vi "校准信息解析.vi"(11 "校准信息":u16[](array[numeric]) caption="关键参数") -> ()   [LabVIEW 2016, in "数据传输系统-02.lvlib"]
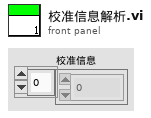
[diagram p1: front panel]
types:
  T1 = cluster{"低标液1浓度":dbl, "低标液1信号值":dbl, "低标液1启用":u16, "低标液2浓度":dbl, "低标液2信号值":dbl, "低标液2启用":u16, "低标液3浓度":dbl, "低标液3信号值":dbl, "低标液3启用":u16, "低标液4浓度":dbl, "低标液4信号值":dbl, "低标液4启用":u16, "低标液5浓度":dbl, "低标液5信号值":dbl, "低标液5启用":u16, "高标液1浓度":dbl, "高标液1信号值":dbl, "高标液1启用":u16, "高标液2浓度":dbl, "高标液2信号值":dbl, "高标液2启用":u16, "高标液3浓度":dbl, "高标液3信号值":dbl, "高标液3启用":u16, "高标液4浓度":dbl, "高标液4信号值":dbl, "高标液4启用":u16, "高标液5浓度":dbl, "高标液5信号值":dbl, "高标液5启用":u16, "低斜率":dbl, "低截距":dbl, "低二次多项式系数":dbl, "低线性相关系数":dbl, "高斜率":dbl, "高截距":dbl, "高二次多项式系数":dbl, "高线性相关系数":dbl}
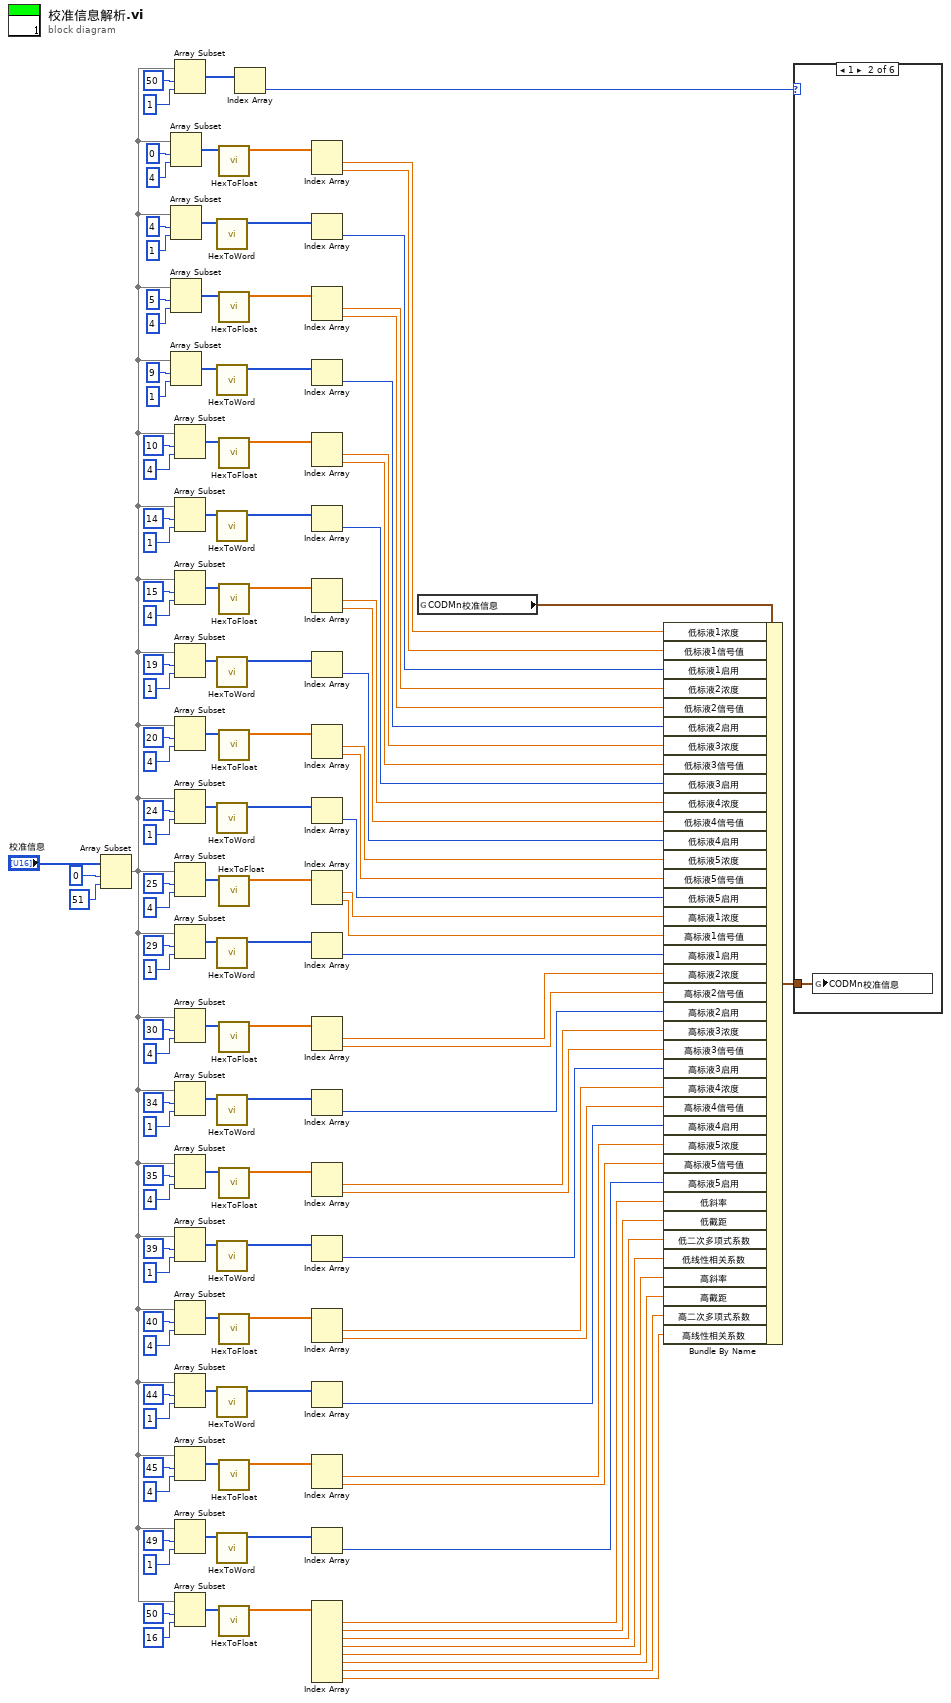
[diagram p0: block diagram]
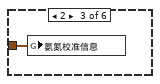
[diagram p3: hidden frame]
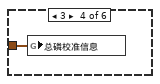
[diagram p4: hidden frame]
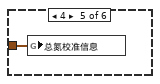
[diagram p5: hidden frame]
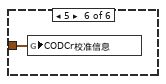
[diagram p6: hidden frame]
diagram:
  n1 = Array Subset(array="校准信息", index=0 ("y"), length=51 ("长度")) -> (w9:u16[])
  n2 = Array Subset(array=w9, index=0 ("索引"), length=4 ("长度")) -> (w126:u16[])
  n3 = Array Subset(array=w9, index=4 ("索引"), length=1 ("长度")) -> (w116:u16[])
  n4 = Array Subset(array=w9, index=5 ("索引"), length=4 ("长度")) -> (w65:u16[])
  n5 = Array Subset(array=w9, index=9 ("索引"), length=1 ("长度")) -> (w66:u16[])
  n6 = Array Subset(array=w9, index=50 ("索引"), length=1 ("长度")) -> (w14:u16[])
  n7 = Array Subset(array=w9, index=10 ("索引"), length=4 ("长度")) -> (w61:u16[])
  n8 = Array Subset(array=w9, index=14 ("索引"), length=1 ("长度")) -> (w60:u16[])
  n9 = Array Subset(array=w9, index=15 ("索引"), length=4 ("长度")) -> (w56:u16[])
  n10 = Array Subset(array=w9, index=19 ("索引"), length=1 ("长度")) -> (w54:u16[])
  n11 = Array Subset(array=w9, index=20 ("索引"), length=4 ("长度")) -> (w47:u16[])
  n12 = Array Subset(array=w9, index=24 ("索引"), length=1 ("长度")) -> (w46:u16[])
  n13 = Array Subset(array=w9, index=25 ("索引"), length=4 ("长度")) -> (w45:u16[])
  n14 = Array Subset(array=w9, index=29 ("索引"), length=1 ("长度")) -> (w44:u16[])
  n15 = Array Subset(array=w9, index=30 ("索引"), length=4 ("长度")) -> (w31:u16[])
  n16 = Array Subset(array=w9, index=34 ("索引"), length=1 ("长度")) -> (w32:u16[])
  n17 = Array Subset(array=w9, index=35 ("索引"), length=4 ("长度")) -> (w28:u16[])
  n18 = Array Subset(array=w9, index=39 ("索引"), length=1 ("长度")) -> (w27:u16[])
  n19 = Array Subset(array=w9, index=40 ("索引"), length=4 ("长度")) -> (w24:u16[])
  n20 = Array Subset(array=w9, index=44 ("索引"), length=1 ("长度")) -> (w23:u16[])
  n21 = Array Subset(array=w9, index=45 ("索引"), length=4 ("长度")) -> (w18:u16[])
  n22 = Array Subset(array=w9, index=49 ("索引"), length=1 ("长度")) -> (w17:u16[])
  n23 = Array Subset(array=w9, index=50 ("索引"), length=16 ("长度")) -> (w13:u16[])
  n24 = call "HexToWord.vi"("数组"=w116) -> ("WORD"=w115:u16[])  [unwired: 10 in]
  n25 = call "HexToWord.vi"("数组"=w66) -> ("WORD"=w113:u16[])  [unwired: 10 in]
  n26 = call "HexToWord.vi"("数组"=w60) -> ("WORD"=w102:u16[])  [unwired: 10 in]
  n27 = call "HexToWord.vi"("数组"=w54) -> ("WORD"=w101:u16[])  [unwired: 10 in]
  n28 = call "HexToWord.vi"("数组"=w46) -> ("WORD"=w92:u16[])  [unwired: 10 in]
  n29 = call "HexToWord.vi"("数组"=w44) -> ("WORD"=w91:u16[])  [unwired: 10 in]
  n30 = call "HexToWord.vi"("数组"=w32) -> ("WORD"=w82:u16[])  [unwired: 10 in]
  n31 = call "HexToWord.vi"("数组"=w27) -> ("WORD"=w81:u16[])  [unwired: 10 in]
  n32 = call "HexToWord.vi"("数组"=w23) -> ("WORD"=w72:u16[])  [unwired: 10 in]
  n33 = call "HexToWord.vi"("数组"=w17) -> ("WORD"=w71:u16[])  [unwired: 10 in]
  n34 = call "HexToFloat.vi"("数组"=w126) -> ("FLOAT"=w125:sgl[])  [unwired: 10 in]
  n35 = call "HexToFloat.vi"("数组"=w65) -> ("FLOAT"=w112:sgl[])  [unwired: 10 in]
  n36 = call "HexToFloat.vi"("数组"=w61) -> ("FLOAT"=w103:sgl[])  [unwired: 10 in]
  n37 = call "HexToFloat.vi"("数组"=w56) -> ("FLOAT"=w100:sgl[])  [unwired: 10 in]
  n38 = call "HexToFloat.vi"("数组"=w47) -> ("FLOAT"=w93:sgl[])  [unwired: 10 in]
  n39 = call "HexToFloat.vi"("数组"=w45) -> ("FLOAT"=w90:sgl[])  [unwired: 10 in]
  n40 = call "HexToFloat.vi"("数组"=w31) -> ("FLOAT"=w83:sgl[])  [unwired: 10 in]
  n41 = call "HexToFloat.vi"("数组"=w28) -> ("FLOAT"=w80:sgl[])  [unwired: 10 in]
  n42 = call "HexToFloat.vi"("数组"=w24) -> ("FLOAT"=w73:sgl[])  [unwired: 10 in]
  n43 = call "HexToFloat.vi"("数组"=w18) -> ("FLOAT"=w70:sgl[])  [unwired: 10 in]
  n44 = call "HexToFloat.vi"("数组"=w13) -> ("FLOAT"=w10:sgl[])  [unwired: 10 in]
  n45 = Index Array(array=w14) -> (element=w118:u16)  [unwired: 1 in]
  n46 = Index Array(array=w125) -> (element #1=w124:sgl, element #2=w123:sgl)  [unwired: 2 in]
  n47 = Index Array(array=w115) -> (element=w114:u16)  [unwired: 1 in]
  n48 = Index Array(array=w112) -> (element #1=w64:sgl, element #2=w63:sgl)  [unwired: 2 in]
  n49 = Index Array(array=w113) -> (element=w62:u16)  [unwired: 1 in]
  n50 = Index Array(array=w103) -> (element #1=w59:sgl, element #2=w58:sgl)  [unwired: 2 in]
  n51 = Index Array(array=w102) -> (element=w57:u16)  [unwired: 1 in]
  n52 = Index Array(array=w100) -> (element #1=w43:sgl, element #2=w42:sgl)  [unwired: 2 in]
  n53 = Index Array(array=w101) -> (element=w41:u16)  [unwired: 1 in]
  n54 = Index Array(array=w93) -> (element #1=w40:sgl, element #2=w39:sgl)  [unwired: 2 in]
  n55 = Index Array(array=w92) -> (element=w38:u16)  [unwired: 1 in]
  n56 = Index Array(array=w90) -> (element #1=w37:sgl, element #2=w36:sgl)  [unwired: 2 in]
  n57 = Index Array(array=w91) -> (element=w35:u16)  [unwired: 1 in]
  n58 = Index Array(array=w83) -> (element #1=w34:sgl, element #2=w33:sgl)  [unwired: 2 in]
  n59 = Index Array(array=w82) -> (element=w30:u16)  [unwired: 1 in]
  n60 = Index Array(array=w80) -> (element #1=w29:sgl, element #2=w26:sgl)  [unwired: 2 in]
  n61 = Index Array(array=w81) -> (element=w25:u16)  [unwired: 1 in]
  n62 = Index Array(array=w73) -> (element #1=w22:sgl, element #2=w21:sgl)  [unwired: 2 in]
  n63 = Index Array(array=w72) -> (element=w20:u16)  [unwired: 1 in]
  n64 = Index Array(array=w70) -> (element #1=w19:sgl, element #2=w16:sgl)  [unwired: 2 in]
  n65 = Index Array(array=w71) -> (element=w15:u16)  [unwired: 1 in]
  n66 = Index Array(array=w10) -> (element #1=w8:sgl, element #2=w7:sgl, element #3=w6:sgl, element #4=w5:sgl, element #5=w4:sgl, element #6=w3:sgl, element #7=w2:sgl, element #8=w1:sgl)  [unwired: 8 in]
  n67 = global read "全局1.vi" "CODMn校准信息"() -> (w117:T1)
  n68 = Bundle By Name(cluster=w117, "低标液1浓度"=w124, "低标液1信号值"=w123, "低标液1启用"=w114, "低标液2浓度"=w64, "低标液2信号值"=w63, "低标液2启用"=w62, "低标液3浓度"=w59, "低标液3信号值"=w58, "低标液3启用"=w57, "低标液4浓度"=w43, "低标液4信号值"=w42, "低标液4启用"=w41, "低标液5浓度"=w40, "低标液5信号值"=w39, "低标液5启用"=w38, "高标液1浓度"=w37, "高标液1信号值"=w36, "高标液1启用"=w35, "高标液2浓度"=w34, "高标液2信号值"=w33, "高标液2启用"=w30, "高标液3浓度"=w29, "高标液3信号值"=w26, "高标液3启用"=w25, "高标液4浓度"=w22, "高标液4信号值"=w21, "高标液4启用"=w20, "高标液5浓度"=w19, "高标液5信号值"=w16, "高标液5启用"=w15, "低斜率"=w8, "低截距"=w7, "低二次多项式系数"=w6, "低线性相关系数"=w5, "高斜率"=w4, "高截距"=w3, "高二次多项式系数"=w2, "高线性相关系数"=w1) -> (w131:T1)
  n69 = case shown="1" w118 {
    tunnel: w131 -> [_ w133 w134 w135 w136 w137]
    frame 0, Default {
    }
    frame 1 {
      n70 = global write "全局1.vi" "CODMn校准信息"(w133) -> ()
    }
    frame 2 {
      n71 = global write "全局1.vi" "氨氮校准信息"(w134) -> ()
    }
    frame 3 {
      n72 = global write "全局1.vi" "总磷校准信息"(w135) -> ()
    }
    frame 4 {
      n73 = global write "全局1.vi" "总氮校准信息"(w136) -> ()
    }
    frame 5 {
      n74 = global write "全局1.vi" "CODCr校准信息"(w137) -> ()
    }
  }
